vi "Servo.vi"() -> ()   [LabVIEW 2018]
uses:
  <vilib>/rvi/Emulation/niFpgaGetClockAttributes.vi
  <vilib>/rvi/Emulation/niFpgaSctlEmulationGetInTimedLoop.vi
  <vilib>/rvi/Emulation/niFpgaEmulationReportErrorSimple.vi
  <vilib>/rvi/eio/common/nirviEmuTemplateMethod_errors.vi
  <vilib>/rvi/Emulation/niFpgaCriticalErrorInLSC.vi
  <vilib>/eio/EIONode/EIONode.xnode
panel:
  in  "Angle [0°;180°]":i16(knob) min=0 max=180 step=1 scale=0.0..180.0
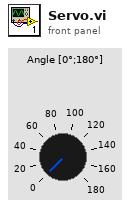
[diagram p1: front panel]
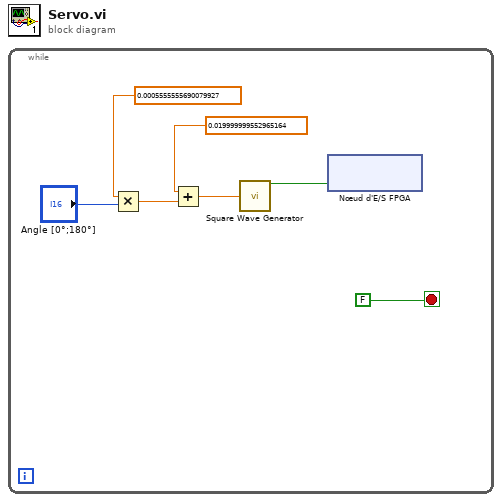
[diagram p0: block diagram]
diagram:
  n1 = while {
    stop <- FALSE stop-if-true
    n2 = Multiply(x=sgl 0.00055555557, y="Angle [0°;180°]") -> (x*y=w4:sgl)
    n3 = Add(x=sgl 0.02, y=w4) -> (x+y=w5:sgl)
    n4 = call "Square Wave Generator"("duty cycle (periods)"=w5) -> ("square wave out"=w7:bool)  [unwired: 14 in]
    n5 = xnode "Nœud d'E/S FPGA"("BB3_DIO0"=w7) -> ()  [unwired: 1 in, 1 out]
  }
